vi "Dynamically Caption Name Update.vi"(8 "error in (no error)":errorcluster, 9 "DUT_Number":string[](array[string]), 10 "Caption Name":string[](array[string]), 11 "Clust Refnum":refnum<vi>) -> (0 "error out":errorcluster)   [LabVIEW 2023, in "GUI.lvlib" / "Diagnostic.lvlib"]
uses:
  Diagnostic.lvlib
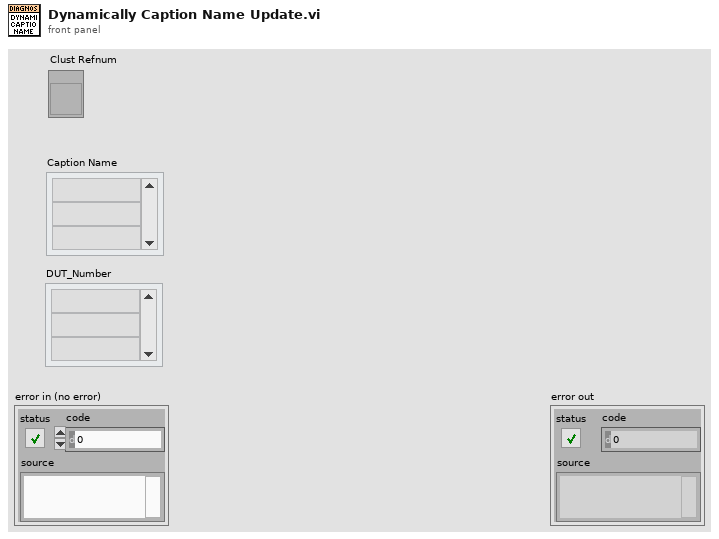
[diagram p1: front panel]
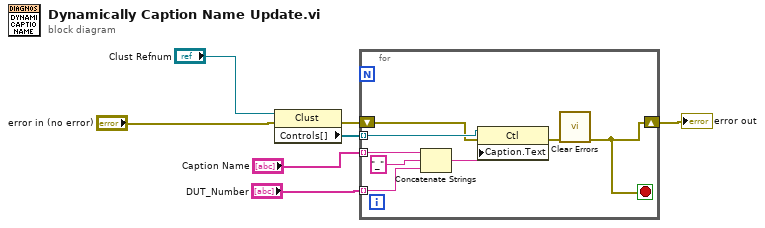
[diagram p0: block diagram]
diagram:
  n1 = property class="Clust"(reference="Clust Refnum", error in="error in (no error)") -> (error out=w5:errorcluster, "Controls[]"=w6:refnum<vi>[])  [unwired: 1 out]
  n2 = for {
    tunnel: w6 -> [w15] mode=indexing
    tunnel: "Caption Name" -> [w13] mode=indexing
    shift-right: [w11] -> w3
    shift-left: w5 -> [w14]
    tunnel: "DUT_Number" -> [w9] mode=indexing
    stop <- w11 stop-if-true
    n3 = Concatenate Strings(w13, "_" ("string"), w9) -> (w10:string)
    n4 = property class="Ctl"(reference=w15, error in=w14, "Caption.Text"=w10) -> (error out=w12:errorcluster)  [unwired: 1 out]
    n5 = call <vilib>:"Clear Errors.vi"("error in (no error)"=w12) -> ("error out"=w11:errorcluster)  [unwired: 5 in, 1 out]
  }
  "error out" <- w3
